vi "LS_372_disable_heater.vi"(6 "Channel":u16, 7 "VISA-Ressourcenname":refnum<visa-resource-name>) -> (3 "Setpoint ist":dbl)   [LabVIEW 2019]
uses:
  Equipment/Lake Shore 372/Lake Shore 372.lvlib
panel:
  in  "Warmup % (50%)":dbl=50.0 min=0.0 max=100.0 step=1.0
  in  "Setpoint Change Delay (25sec)":i32=25 min=1 max=255 step=1
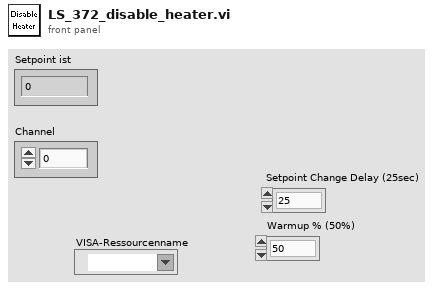
[diagram p1: front panel]
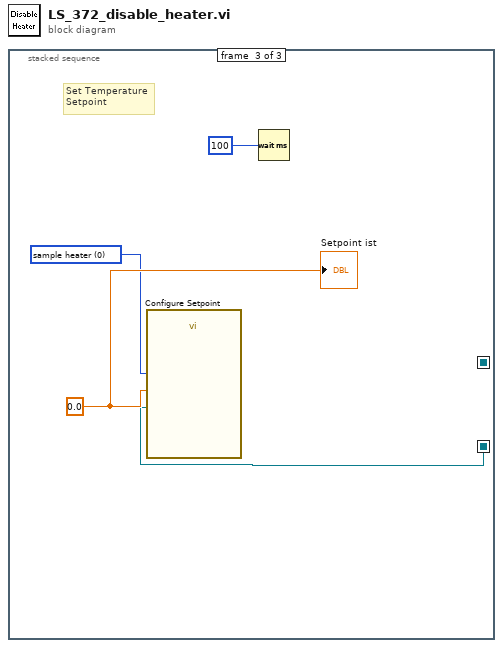
[diagram p0: block diagram]
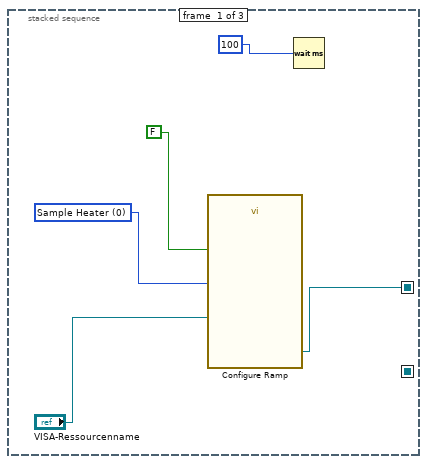
[diagram p2: hidden frame]
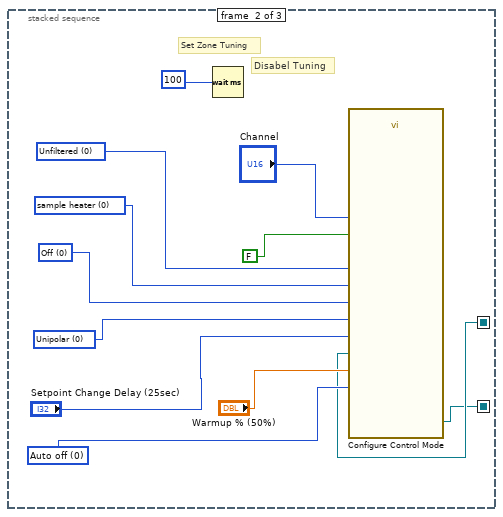
[diagram p3: hidden frame]
diagram:
  n1 = stacked-sequence {
    seq-local: [w2 _ _] -> [_ w7 _]
    seq-local: [_ w6 _] -> [_ _ w20]
    frame #0 {
      w4 = u16 0 items=["Sample Heater ", "Warm-up Heater "] ("Output (0: Sample Heater)")
      n2 = call "Configure Ramp.vi"("Enable Ramping (F: Disable)"=FALSE, "Output (0: Sample Heater)"=w4, "VISA resource name"="VISA-Ressourcenname") -> ("VISA resource name out"=w2:refnum<visa-resource-name>)  [unwired: 7 in, 1 out]
      n3 = Wait (ms)(milliseconds to wait=100) -> ()  [unwired: 1 out]
    }
    frame #1 {
      w11 = u16 0 items=["Auto off", "Continuous"] ("Warmup Control (0: Auto off)")
      w13 = u16 0 items=["Unfiltered", "Filtered"] ("Filtered Readings (0: Unfiltered)")
      w15 = u16 0 items=["Unipolar", "Bipolar"] ("Polarity (0: Unipolar)")
      w16 = u16 0 items=["sample heater", "output 1 (warm-up heater) ", "output 2 (analog/still)"] ("Output (0: sample heater)")
      w17 = u16 0 items=["Off", "Monitor Out", "Open Loop (Manual)", "Zone", "Still", "Closed Loop (PID)", "Warm-up"] ("Output Mode (0: Off)")
      # "Set Zone Tuning"
      # "Disabel Tuning"
      n4 = Wait (ms)(milliseconds to wait=100) -> ()  [unwired: 1 out]
      n5 = call "Configure Control Mode.vi"("VISA resource name"=w7, "Enable Power-up (F: Disable)"=FALSE, "Setpoint Change Delay (25sec)"="Setpoint Change Delay (25sec)", "Output (0: sample heater)"=w16, "Channel (1:1)"="Channel", "Output Mode (0: Off)"=w17, "Polarity (0: Unipolar)"=w15, "Filtered Readings (0: Unfiltered)"=w13, "Warmup Control (0: Auto off)"=w11, "Warmup % (50%)"="Warmup % (50%)") -> ("VISA resource name out"=w6:refnum<visa-resource-name>)  [unwired: 4 in, 1 out]
    }
    frame #2 {
      w18 = u16 0 items=["sample heater", "output 1 (warm-up heater) ", "output 2 (analog/still)"] ("Output (0: sample heater)")
      w21 = 0.0
      # "Set Temperature\nSetpoint"
      n6 = call "Configure Setpoint.vi"("Setpoint (0.00000E+0)"=w21, "Output (0: Sample Heater)"=w18, "VISA resource name"=w20) -> ()  [unwired: 7 in, 2 out]
      n7 = Wait (ms)(milliseconds to wait=100) -> ()  [unwired: 1 out]
      "Setpoint ist" <- w21
    }
  }
